vi "7 đèn .vi"() -> ()   [LabVIEW 2020]
panel:
  in  "stop":bool
  in  "Numeric 3":dbl
  out "Numeric 2":dbl
  in  "Numeric":dbl
  out "Boolean 7":bool
  out "Boolean 6":bool
  out "Boolean 5":bool
  out "Boolean 4":bool
  out "Boolean 3":bool
  out "Boolean 2":bool
  out "Boolean":bool
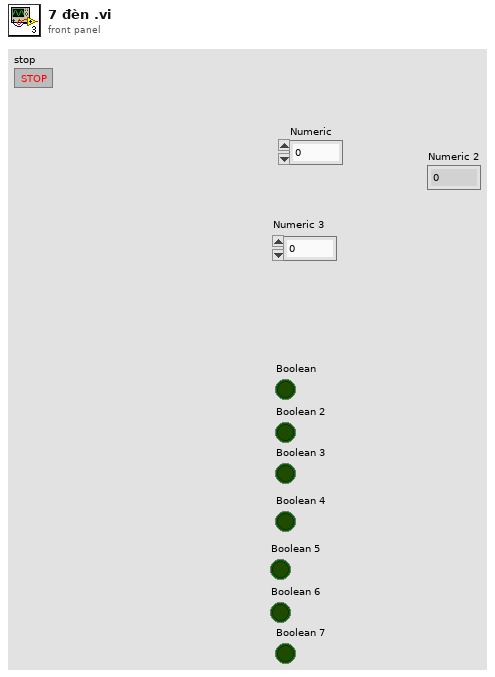
[diagram p1: front panel]
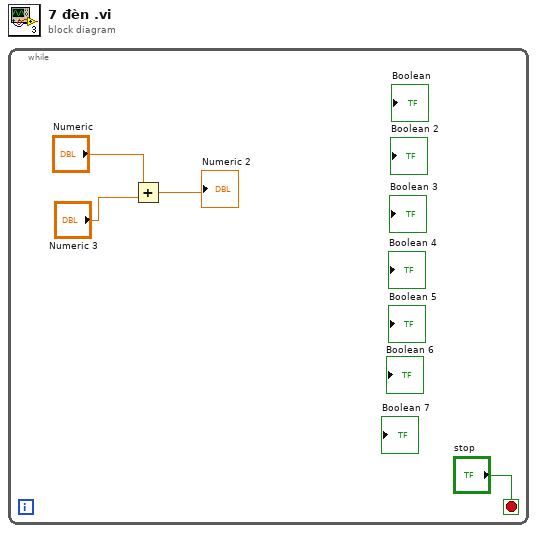
[diagram p0: block diagram]
diagram:
  n1 = while {
    stop <- "stop" stop-if-true
    n2 = Add(x="Numeric", y="Numeric 3") -> (x+y=→"Numeric 2":dbl)
  }
